vi "FlowControl2.vi"() -> ()   [LabVIEW 2016]
uses:
  <userlib>/Fluigent/Fluigent MFCS/FluigentMFCS_Full.llb/MFCS_EZ Detect.vi
  <userlib>/Fluigent/Fluigent MFCS/FluigentMFCS_Full.llb/MFCS_EZ Initialization.vi
  <userlib>/Fluigent/Fluigent MFCS/FluigentMFCS_Full.llb/MFCS_EZ Read All Channels Pressure.vi
  <userlib>/Fluigent/Fluigent MFCS/FluigentMFCS_Full.llb/MFCS_EZ Write Channel Pressure.vi
  <userlib>/Fluigent/Fluigent MFCS/FluigentMFCS_Full.llb/MFCS_EZ Close.vi
panel:
  in  "Pressure Setpoints":dbl[](array[numeric])
  out "All Channels Pressure":dbl[](array[numeric])
  out "error out":errorcluster
  out "Waveform Chart":waveform(dbl)[](graph)
  out "Flow Rates":dbl[](array[numeric])
  in  "stop":bool
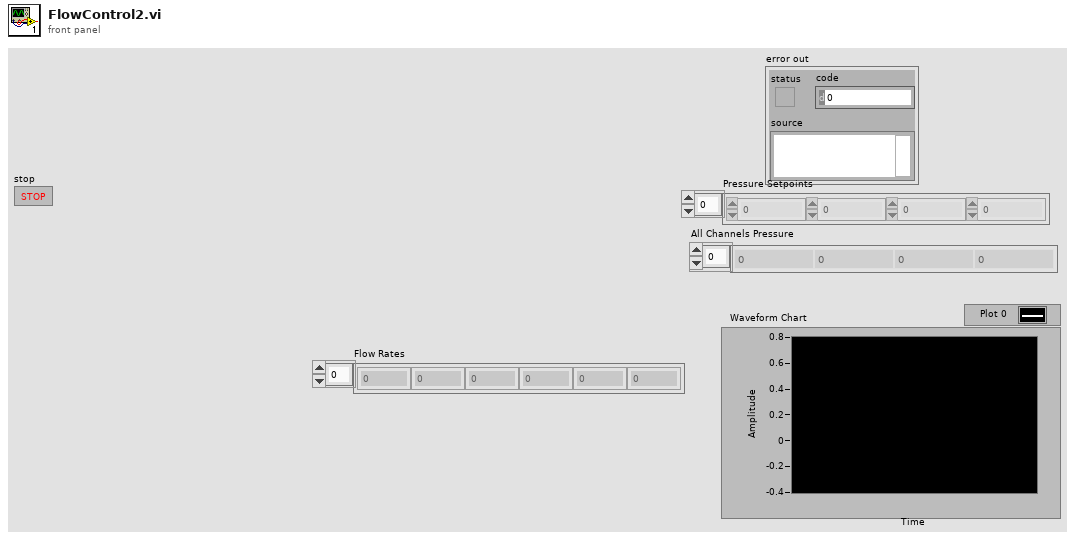
[diagram p1: front panel]
types:
  T1 = typedef "_EZmfcsSN.ctl" = u16
  T2 = typedef "_frpRefNum" = refnum<k1>
  T3 = typedef "_EZmfcsRefNum.ctl" = refnum<k1>
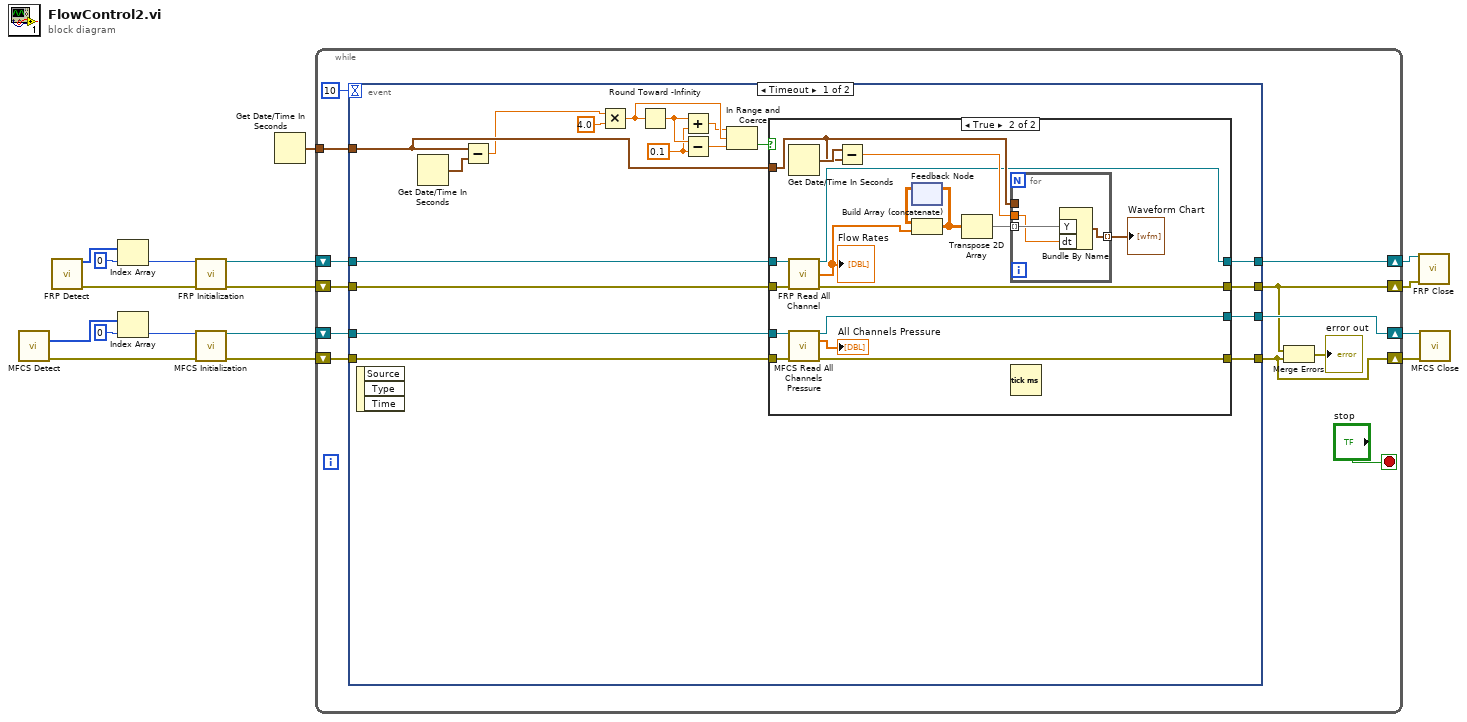
[diagram p0: block diagram]
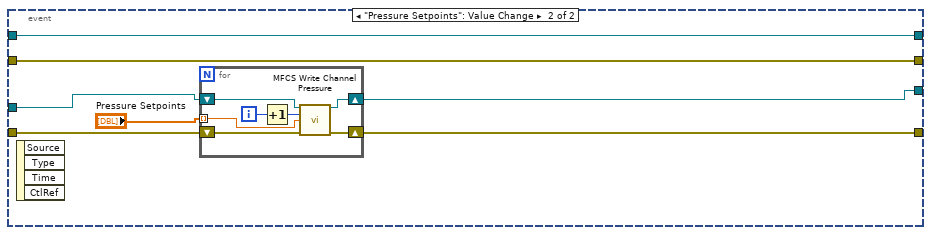
[diagram p3: hidden frame]
diagram:
  n1 = call-poly <userlib>:"MFCS Detect.vi"() -> ("[SN MFCS_EZ]"=w17:T1[], "error out"=w15:errorcluster)  [unwired: 14 in]
  n2 = call <userlib>:"FRP Detect.vi"() -> ("FLOWBOARD List"=w14:u16[], "error out"=w11:errorcluster)  [unwired: 14 in]
  n3 = Index Array(array=w14, index=0) -> (element=w10:u16)
  n4 = Index Array(array=w17, index=0) -> (element=w16:T1)
  n5 = call <userlib>:"FRP Initialization.vi"("Serial Number"=w10, "error in (no error)"=w11) -> ("FRP out"=w9:T2, "error out"=w7:errorcluster)  [unwired: 11 in, 1 out]
  n6 = call-poly <userlib>:"MFCS Initialization.vi"("SN MFCS_EZ"=w16, "error in (no error)"=w15) -> ("MFCS_EZ"=w8:T3, "error out"=w6:errorcluster)  [unwired: 11 in, 1 out]
  n7 = Get Date/Time In Seconds() -> (seconds since 1Jan1904=w3:timestamp)
  n8 = while {
    shift-right: [w20] -> w1
    shift-left: w7 -> [w21]
    shift-right: [w23] -> w2
    shift-left: w9 -> [w24]
    shift-right: [w19] -> w4
    shift-left: w6 -> [w26]
    shift-right: [w22] -> w5
    shift-left: w8 -> [w27]
    tunnel: w3 -> [w25]
    stop <- "stop" stop-if-true
    n9 = event shown="[0] Timeout" {
      selector: _ -> [_ _]
      dyn-events: _ -> [_ _]
      timeout: 10 -> [_ _]
      tunnel: w27 -> [w45 w77]
      tunnel: [w44 w76] -> w22
      tunnel: [w32 w73] -> w20
      tunnel: [w43 w75] -> w19
      tunnel: w26 -> [w37 w74]
      tunnel: w25 -> [w35 _]
      tunnel: w24 -> [w34 w72]
      tunnel: [w33 w72] -> w23
      tunnel: w21 -> [w31 w73]
      event Timeout {
        w40 = 0.1 ("floor(x): largest int <= x")
        n10 = event-data() -> ()  [unwired: 1 in, 3 out]
        n11 = Get Date/Time In Seconds() -> (seconds since 1Jan1904=w36:timestamp)
        n12 = Subtract(x=w35, y=w36) -> (x-y=w30:dbl)
        n13 = Multiply(x=w30, y=4.0) -> (x*y=w42:dbl)
        n14 = Round Toward -Infinity(1:w42) -> (0:w41:dbl)
        n15 = Add(x=w41, y=w40) -> (x+y=w39:dbl)
        n16 = Subtract(x=w41, y=w40) -> (x-y=w38:dbl)
        n17 = In Range and Coerce(upper limit=w39, x=w42, lower limit=w38) -> (In Range?=w46:bool)  [unwired: 1 out]
        n18 = case shown="True" w46 {
          tunnel: w45 -> [w51 w68]
          tunnel: [w51 w67] -> w44
          tunnel: w37 -> [w50 w66]
          tunnel: [w50 w65] -> w43
          tunnel: w35 -> [_ w59]
          tunnel: w34 -> [w49 w58]
          tunnel: [w49 w57] -> w33
          tunnel: [w48 w55] -> w32
          tunnel: w31 -> [w48 w54]
          frame False {
          }
          frame True {
            n19 = Get Date/Time In Seconds() -> (seconds since 1Jan1904=w61:timestamp)
            n20 = call <userlib>:"FRP Read All Channel.vi"("FRP"=w58, "error in (no error)"=w54) -> ("FRP out"=w57:T2, "All Flow-Rates"=w56:dbl[], "error out"=w55:errorcluster)  [unwired: 11 in]
            "Flow Rates" <- w56
            n21 = call-poly <userlib>:"MFCS Read All Channels Pressure.vi"("MFCS_EZ"=w68, "error in (no error)"=w66) -> ("MFCS_EZ out"=w67:T3, "All Channels Pressure"=→"All Channels Pressure":dbl[], "error out"=w65:errorcluster)  [unwired: 11 in]
            n22 = Subtract(x=w61, y=w59) -> (x-y=w60:dbl)
            n23 = feedback #1() -> (w63:dbl[][])  [unwired: 1 in]
            n24 = Build Array (concatenate)(w63, w56) -> (w62:dbl[][])
            n25 = feedback-in #1(w62) -> ()
            n26 = Transpose 2D Array(2D array=w62) -> (transposed array=w53:dbl[][])
            n27 = for {
              tunnel: w59 -> [_]
              tunnel: w60 -> [w69]
              tunnel: w53 -> [w71] mode=indexing
              tunnel: [w70] -> w52 mode=indexing
              n28 = Bundle By Name("Y"=w71, "dt"=w69) -> (w70:waveform(dbl))  [unwired: 1 in]
            }
            "Waveform Chart" <- w52
            n29 = Tick Count (ms)() -> ()  [unwired: 1 out]
          }
        }
      }
      event "Pressure Setpoints": Value Change {
        n30 = event-data() -> ()  [unwired: 1 in, 4 out]
        n31 = for {
          tunnel: "Pressure Setpoints" -> [w85] mode=indexing
          shift-right: [w82] -> w76
          shift-left: w77 -> [w83]
          shift-right: [w80] -> w75
          shift-left: w74 -> [w81]
          i -> [w84]
          n32 = Increment(x=w84) -> (x+1=w79:i32)
          n33 = call-poly <userlib>:"MFCS Write Channel Pressure.vi"("MFCS_EZ"=w83, "Channel Number (default=1)"=w79, "Pressure (mBar)"=w85, "error in (no error)"=w81) -> ("MFCS_EZ out"=w82:T3, "error out"=w80:errorcluster)  [unwired: 10 in]
        }
      }
    }
    n34 = Merge Errors(w20, w19) -> (→"error out":errorcluster)
  }
  n35 = call <userlib>:"FRP Close.vi"("FRP"=w2, "error in (no error)"=w1) -> ()  [unwired: 13 in, 1 out]
  n36 = call-poly <userlib>:"MFCS Close.vi"("MFCS_EZ"=w5, "error in (no error)"=w4) -> ()  [unwired: 13 in, 1 out]
